vi "Export PID Parameters.vi"(8 "error in":errorcluster, 10 "Parameters":dbl[][](array[numeric]), 11 "Control Loop":string) -> (0 "error out":errorcluster)   [LabVIEW 2019, in "Control Addon Shared.lvlib"]
uses:
  Control Addon Shared.lvlib
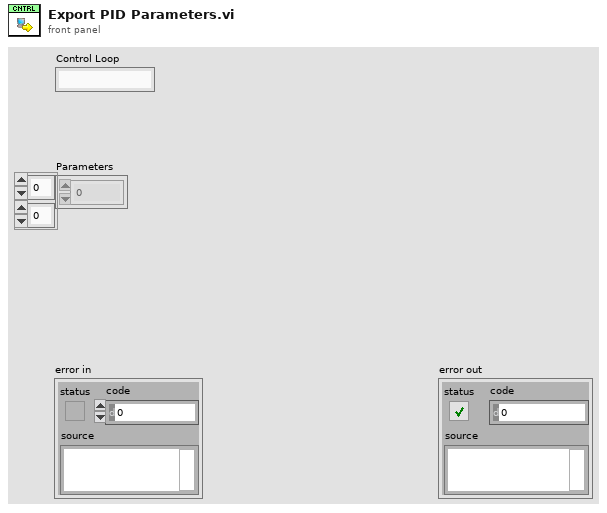
[diagram p1: front panel]
types:
  T1 = enum16{"open", "replace", "create", "open or create", "replace or create", "replace or create with confirmation"}
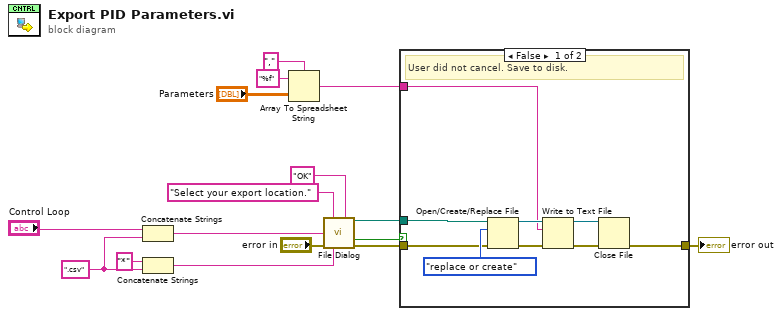
[diagram p0: block diagram]
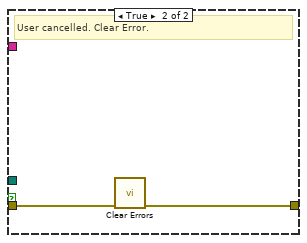
[diagram p2: hidden frame]
diagram:
  w14 = ".csv" ("pattern (all files)")
  n1 = Concatenate Strings("Control Loop", w14) -> (w13:string)
  n2 = Concatenate Strings("*" ("pattern (all files)"), w14) -> (w16:string)
  n3 = Array To Spreadsheet String(delimiter (Tab)=",", array="Parameters", 3:"%f" ("format string")) -> (spreadsheet string=w8:string)
  n4 = call "File Dialog"("prompt"="Select your export location.", "button label"="OK", "default name"=w13, "error in"="error in", "pattern (all files)"=w16) -> ("selected path"=w7:path, "cancelled"=w11:bool, "error out"=w12:errorcluster)  [unwired: 7 in, 1 out]
  n5 = case shown="False" w11 {
    tunnel: w7 -> [w25 _]
    tunnel: w8 -> [w20 _]
    tunnel: w12 -> [w18 w27]
    tunnel: [w17 w26] -> w2
    frame False {
      # "User did not cancel. Save to disk."
      n6 = Open/Create/Replace File(file path (use dialog)=w25, error in=w18, operation (0:open)=T1."replace or create") -> (refnum out=w24:refnum<file>, error out=w21:errorcluster)  [unwired: 3 in, 1 out]
      n7 = Write to Text File(file (use dialog)=w24, text=w20, error in=w21) -> (refnum out=w22:refnum<file>, error out=w23:errorcluster)  [unwired: 1 in, 1 out]
      n8 = Close File(refnum=w22, error in=w23) -> (error out=w17:errorcluster)  [unwired: 1 out]
    }
    frame True {
      # "User cancelled. Clear Error."
      n9 = call <vilib>:"Clear Errors.vi"("error in (no error)"=w27) -> ("error out"=w26:errorcluster)  [unwired: 5 in, 1 out]
    }
  }
  "error out" <- w2
